vi "Clamp.vi"() -> ()   [LabVIEW 2014]
doc: "This example illustrates the use of the horizontal clamp tool. You can draw a region of inspection that contains at least two edges in the image. The VI measures the distance between the first and last edges."
uses:
  <vilib>/vision/NI_Vision_Development_Module.lvlib
panel:
  out "Distance (pixels)":sgl
  out "Image":T1(plugin-control)
  in  "Stop":bool
  # "Overview: Demonstrates how to use the IMAQ Clamp Horizontal Max function to find the maximum horizontal distance between edges found in the Region of Interest.\nRequirements: Vision Development Software.\nInstructions:\n1. Run the VI.\n2. Draw a Region of Interest in the image containing at least 2 edges to calculate the maximum horizontal distance."
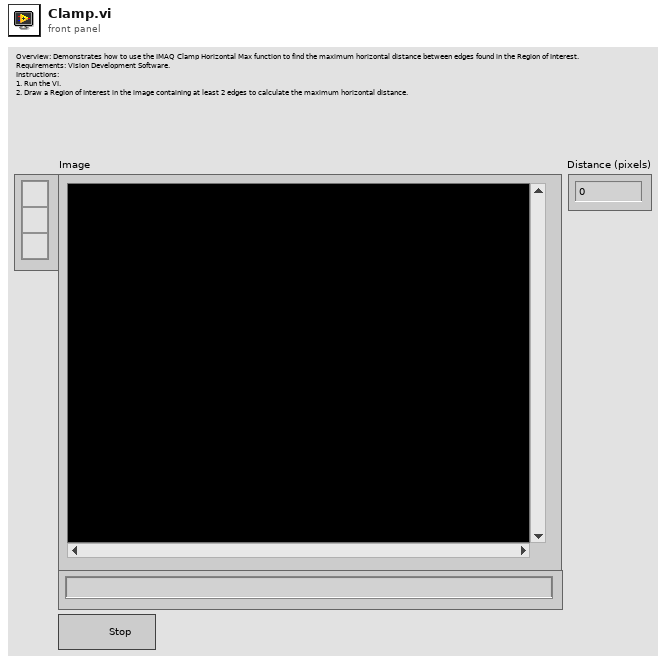
[diagram p1: front panel]
types:
  T1 = typedef "IMAQ Image.ctl" = refnum<image>
  T2 = typedef "IMAQ Rectangle" = cluster{"Left":i32, "Top":i32, "Right":i32, "Bottom":i32, "Rotation":dbl}
  T3 = typedef "ROI Descriptor" = cluster{"Global Rectangle":i32[], "Contours":cluster{"ID":enum32{"External", "Internal"}, "Type":u32, "Coordinates":i32[]}[]}
  T4 = cluster{"Contrast":i32, "Filter width":i32, "Steepness":i32, "Subsampling Ratio":u32, "Show Search Area":bool, "Show Search Lines":bool, "Show Edges Found":bool, "Show Result":bool}
  T5 = cluster{"Global Rectangle":i32[], "Contours":cluster{"Contour Type":u32, "ROI Type":u32, "Points":i32[]}[]}
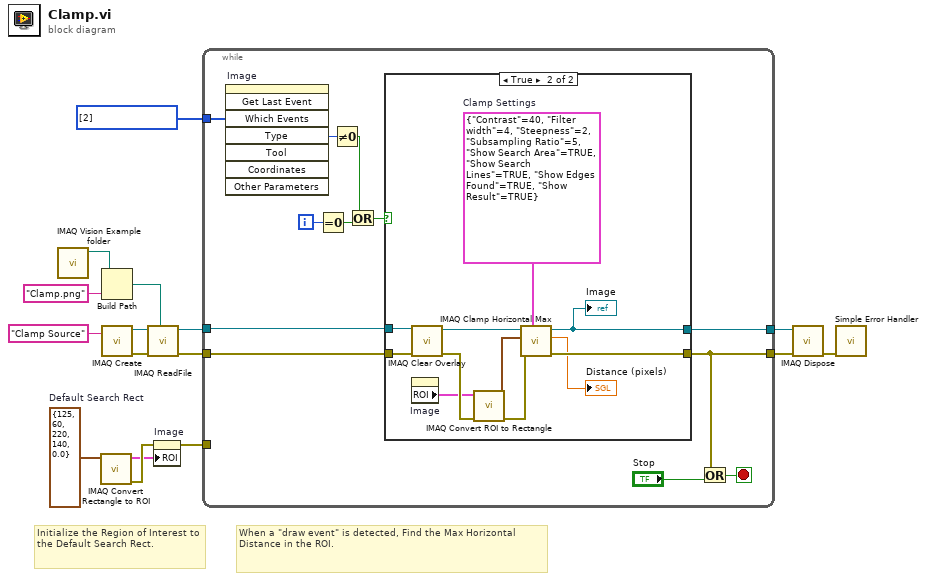
[diagram p0: block diagram]
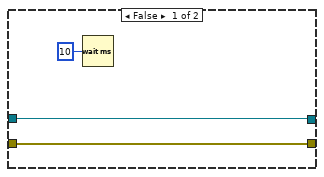
[diagram p2: hidden frame]
diagram:
  w5 = i32[] [2] items=["No  event", "Click event", "Draw event", "Move event", "Size event", "Scroll event", "Activate event", "Close event", "Double click event"] ("Events list (all)")
  w4 = T2 {"Left"=125, "Top"=60, "Right"=220, "Bottom"=140, "Rotation"=0.0}  # Default Search Rect
  # "When a \"draw event\" is detected, Find the Max Horizontal Distance in the ROI."
  # "Initialize the Region of Interest to the Default Search Rect."
  n1 = call "IMAQ Vision Example folder.vi"() -> ("Example Image Path"=w14:path)  [unwired: 11 in]
  n2 = call "IMAQ Convert Rectangle to ROI"("Rectangle"=w4) -> ("error out"=w3:errorcluster, "ROI Descriptor"=w2:T3)  [unwired: 8 in]
  n3 = Build Path(base path=w14, name or relative path="Clamp.png") -> (appended path=w11:path)
  n4 = call "IMAQ Create"("Image Name"="Clamp Source") -> ("New Image"=w15:T1, "error out"=w13:errorcluster)  [unwired: 4 in]
  n5 = call "IMAQ ReadFile"("File Path"=w11, "error in (no error)"=w13, "Image"=w15) -> ("error out"=w6:errorcluster, "Image Out"=w7:T1)  [unwired: 4 in, 3 out]
  n6 = property on="Image" class="ImageControl"(error in=w3, "ROI"=w2) -> (error out=w1:errorcluster)  [unwired: 1 in, 1 out]
  n7 = while {
    tunnel: w7 -> [w28]
    tunnel: [w18] -> w9
    tunnel: [w26] -> w8
    tunnel: w6 -> [w25]
    tunnel: w5 -> [w24]
    tunnel: w1 -> [_]
    i -> [w23]
    stop <- w17 stop-if-true
    n8 = invoke on="Image" class="ImageControl" method="Get Last Event"("Which Events"=w24) -> ("Type"=w27:i32)  [unwired: 7 in, 7 out]
    n9 = Equal To 0?(x=w23) -> (x = 0?=w22:bool)
    n10 = Not Equal To 0?(x=w27) -> (x != 0?=w21:bool)
    n11 = Or(x=w21, y=w22) -> (x .or. y?=w20:bool)
    n12 = case shown="True" w20 {
      tunnel: w28 -> [w29 w35]
      tunnel: [w30 w40] -> w18
      tunnel: [w29 w39] -> w26
      tunnel: w25 -> [w30 w38]
      frame False {
        n13 = Wait (ms)(milliseconds to wait=u32 10) -> ()  [unwired: 1 out]
      }
      frame True {
        w41 = T4 {"Contrast"=40, "Filter width"=4, "Steepness"=2, "Subsampling Ratio"=5, "Show Search Area"=TRUE, "Show Search Lines"=TRUE, "Show Edges Found"=TRUE, "Show Result"=TRUE}  # Clamp Settings
        n14 = call "IMAQ Clear Overlay"("error in (no error)"=w38, "Image"=w35) -> ("error out"=w34:errorcluster, "Image Out"=w42:T1)  [unwired: 8 in]
        n15 = property on="Image" class="ImageControl"() -> ("ROI"=w32:T5)  [unwired: 2 in, 2 out]
        n16 = call "IMAQ Convert ROI to Rectangle"("error in (no error)"=w34, "ROI Descriptor"=w32) -> ("error out"=w33:errorcluster, "Rectangle"=w37:T2)  [unwired: 7 in]
        n17 = call "IMAQ Clamp Horizontal Max"("Settings"=w41, "error in (no error)"=w33, "Rectangle"=w37, "Image"=w42) -> ("error out"=w40:errorcluster, "Distance"=→"Distance (pixels)":sgl, "Image Out"=w39:T1)  [unwired: 3 in, 2 out]
        "Image" <- w39
      }
    }
    n18 = Or(x=w18, y="Stop") -> (x .or. y?=w17:bool)
  }
  n19 = call "IMAQ Dispose"("Image"=w8, "error in (no error)"=w9) -> ("error out"=w16:errorcluster)  [unwired: 4 in]
  n20 = call <vilib>:"Simple Error Handler.vi"("error in (no error)"=w16) -> ()  [unwired: 4 in, 5 out]
